vi "Pathhorafech(SubVI).vi"() -> (0 "path":path)   [LabVIEW 2015]
panel:
  out "date/time string":string
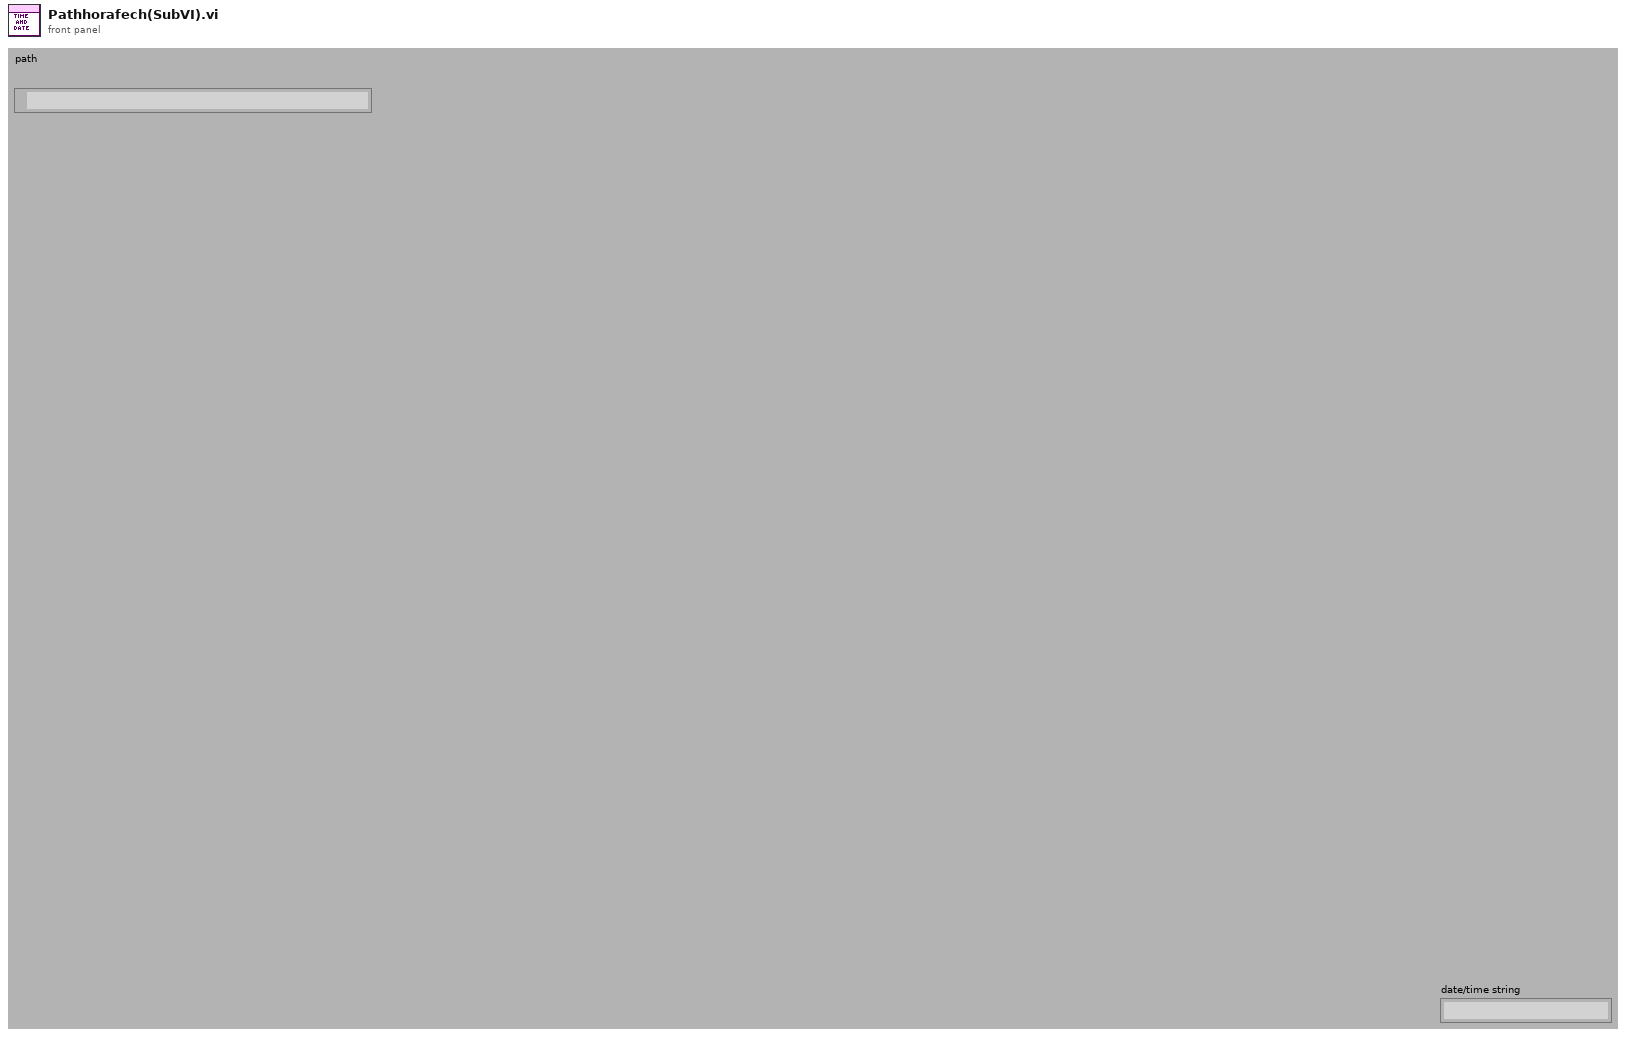
[diagram p1: front panel]
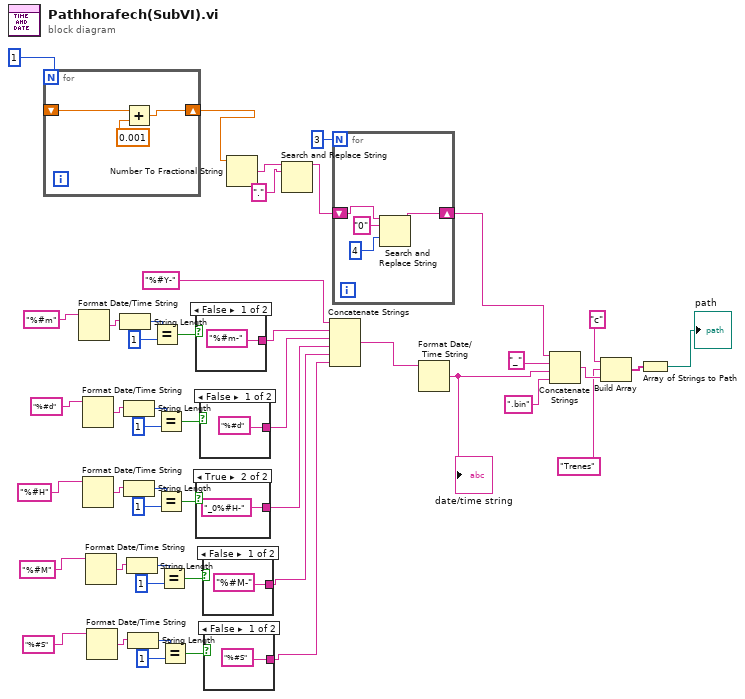
[diagram p0: block diagram]
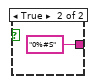
[diagram p2: hidden frame]
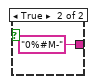
[diagram p3: hidden frame]
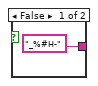
[diagram p4: hidden frame]
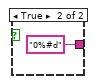
[diagram p5: hidden frame]
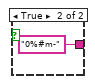
[diagram p6: hidden frame]
diagram:
  n1 = for {
    N: 1 -> [_]
    shift-right: [w50] -> w42
    shift-left: _ -> [w48]
    n2 = Add(x=w48, y=0.001) -> (x+y=w50:dbl)
  }
  n3 = Format Date/Time String(time format string (%c)="%#m") -> (date/time string=w29:string)  [unwired: 2 in]
  n4 = Format Date/Time String(time format string (%c)="%#d") -> (date/time string=w34:string)  [unwired: 2 in]
  n5 = Format Date/Time String(time format string (%c)="%#H") -> (date/time string=w16:string)  [unwired: 2 in]
  n6 = Format Date/Time String(time format string (%c)="%#M") -> (date/time string=w11:string)  [unwired: 2 in]
  n7 = Format Date/Time String(time format string (%c)="%#S") -> (date/time string=w6:string)  [unwired: 2 in]
  n8 = String Length(string=w29) -> (length=w30:i32)
  n9 = String Length(string=w34) -> (length=w35:i32)
  n10 = String Length(string=w16) -> (length=w17:i32)
  n11 = String Length(string=w11) -> (length=w12:i32)
  n12 = String Length(string=w6) -> (length=w7:i32)
  n13 = Equal?(x=w30, y=1) -> (x = y?=w32:bool)
  n14 = Equal?(x=w35, y=1) -> (x = y?=w37:bool)
  n15 = Equal?(x=w17, y=1) -> (x = y?=w19:bool)
  n16 = Equal?(x=w12, y=1) -> (x = y?=w14:bool)
  n17 = Equal?(x=w7, y=1) -> (x = y?=w9:bool)
  n18 = case shown="False" w32 {
    tunnel: ["%#m-" ("time format string (%c)") "0%#m-" ("time format string (%c)")] -> w39
    frame False {
    }
    frame True {
    }
  }
  n19 = case shown="True" w19 {
    tunnel: ["_%#H-" ("time format string (%c)") "_0%#H-" ("time format string (%c)")] -> w4
    frame False {
    }
    frame True {
    }
  }
  n20 = case shown="False" w37 {
    tunnel: ["%#d" ("time format string (%c)") "0%#d" ("time format string (%c)")] -> w40
    frame False {
    }
    frame True {
    }
  }
  n21 = case shown="False" w14 {
    tunnel: ["%#M-" ("time format string (%c)") "0%#M-" ("time format string (%c)")] -> w3
    frame False {
    }
    frame True {
    }
  }
  n22 = case shown="False" w9 {
    tunnel: ["%#S" ("time format string (%c)") "0%#S" ("time format string (%c)")] -> w2
    frame False {
    }
    frame True {
    }
  }
  n23 = Number To Fractional String(number=w42) -> (F-format string=w46:string)  [unwired: 3 out]
  n24 = Search and Replace String(input string=w46, search string="." ("replace string (\"\")")) -> (result string=w44:string)  [unwired: 1 in, 8 out]
  n25 = Concatenate Strings("%#Y-" ("time format string (%c)"), w39, w40, w4, w3, w2) -> (w41:string)
  n26 = for {
    N: 3 -> [_]
    shift-right: [w63] -> w1
    shift-left: w44 -> [w61]
    n27 = Search and Replace String(input string=w61, search string="0", offset=4 ("offset (0)")) -> (result string=w63:string)  [unwired: 1 in, 7 out]
  }
  n28 = Format Date/Time String(time format string (%c)=w41) -> (date/time string=w21:string)  [unwired: 2 in]
  "date/time string" <- w21
  n29 = Concatenate Strings(w1, "_" ("replace string (\"\")"), w21, ".bin" ("string")) -> (w27:string)
  n30 = Build Array("c", "Trenes" ("element"), w27) -> (w26:string[])
  n31 = Array of Strings to Path(0:w26) -> (2:→"path":path)  [unwired: 1 out]
